vi "Initialize.vi"(8 "error in":errorcluster, 11 "Ballard ARINC-429 shared resources in":refnum<class "Shared Resources.lvclass">) -> (0 "error out":errorcluster, 3 "Ballard ARINC-429 shared resources out":refnum<class "Shared Resources.lvclass">)   [LabVIEW 2020, in "Ballard ARINC 429 Engine.lvlib" / "Implementation.lvlib" / "Shared Resources.lvclass"]
uses:
  Shared Resources.lvclass
  Custom Device/Custom Device.lvlib
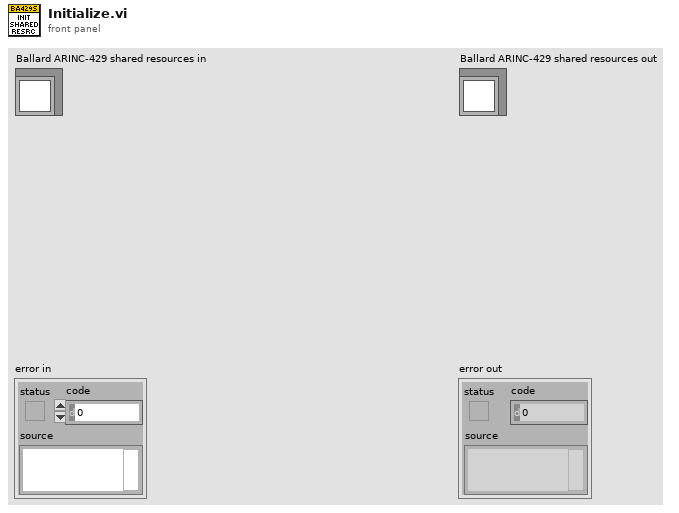
[diagram p1: front panel]
types:
  T1 = typedef "Device Parameters.ctl" = cluster{"initialization method":T2, "card number":i32, "PXI slot number":i32, "core number":i32}
  T2 = typedef "Initialization Method.ctl" = enum16{"PXI Slot Number", "Card Number"}
  T3 = typedef "Ballard ARINC 429 Engine.lvlib/Custom Device.lvlib/Logging Configuration.ctl" = cluster{"configured":bool, "directory":string}
  T4 = typedef "Ballard ARINC 429 Engine.lvlib/Custom Device.lvlib/Hardware Handles.ctl" = cluster{"core handle":u64, "core reader handle":u64, "channel handles":u64[]}
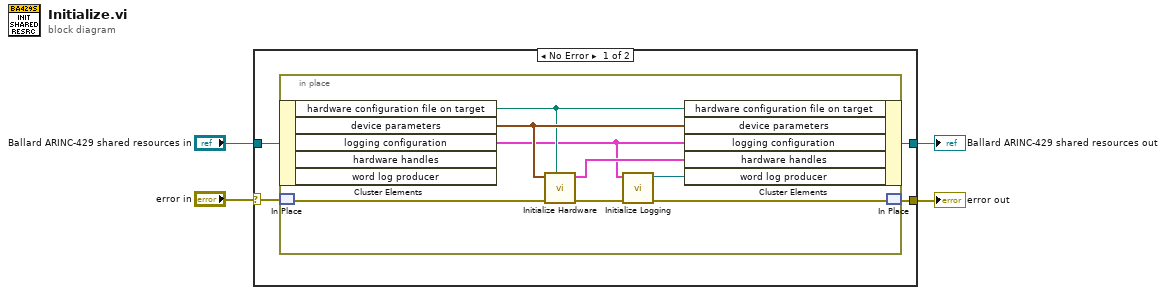
[diagram p0: block diagram]
diagram:
  n1 = case shown="No Error" "error in" {
    selector: "error in" -> [w8 w17]
    tunnel: "Ballard ARINC-429 shared resources in" -> [w6 w18]
    tunnel: [w7 w17] -> w2
    tunnel: [w5 w18] -> w1
    frame No Error {
      n2 = in-place {
        n3 = in-place-cluster #1(w6) -> ("hardware configuration file on target"=w14:path, "device parameters"=w15:T1, "logging configuration"=w9:T3)  [unwired: 2 out]
        n4 = in-place-match #2(w8) -> (w13:errorcluster)
        n5 = call "Initialize Hardware.vi"("RT config file"=w14, "error in"=w13, "device parameters"=w15) -> ("error out"=w12:errorcluster, "RT handles"=w16:T4)  [unwired: 6 in, 1 out]
        n6 = call "Initialize Logging.vi"("error in (no error)"=w12, "logging configuration"=w9) -> ("error out"=w11:errorcluster, "Producer"=w10:refnum<class "Word Log Producer.lvclass">)  [unwired: 8 in]
        n7 = in-place-cluster #1("hardware configuration file on target"=w14, "device parameters"=w15, "logging configuration"=w9, "hardware handles"=w16, "word log producer"=w10) -> (w5:refnum<class "Shared Resources.lvclass">)
        n8 = in-place-match #2(w11) -> (w7:errorcluster)
      }
    }
    frame Error {
    }
  }
  "error out" <- w2
  "Ballard ARINC-429 shared resources out" <- w1
